vi "WID to Tree Data.vi"(11 "WID":string) -> (1 "Worker Tree Depth":i32, 2 "Alias":string, 3 "Owner WID":string)   [LabVIEW 2017, in "Application Manager.lvclass"]
uses:
  Application Manager.lvclass
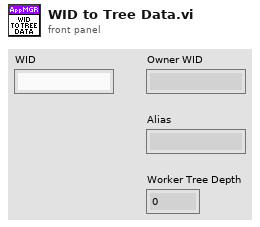
[diagram p1: front panel]
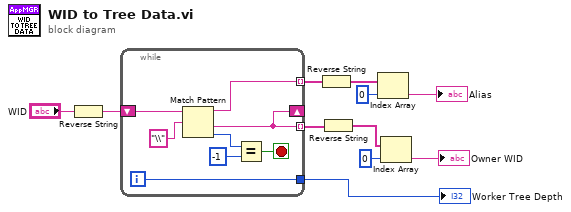
[diagram p0: block diagram]
diagram:
  n1 = Reverse String(1:"WID") -> (0:w10:string)
  n2 = while {
    shift-right: [w13] -> _
    shift-left: w10 -> [w19]
    tunnel: [w14] -> w9 mode=indexing
    tunnel: [w13] -> w3 mode=indexing
    tunnel: [w12] -> w1
    i -> [w12]
    stop <- w15 stop-if-true
    n3 = Match Pattern(string=w19, regular expression="\\") -> (before substring=w14:string, after substring=w13:string, offset past match=w17:i32)  [unwired: 1 in, 1 out]
    n4 = Equal?(x=w17, y=-1) -> (x = y?=w15:bool)
  }
  "Worker Tree Depth" <- w1
  n5 = Reverse String(1:w9) -> (0:w6:string[])
  n6 = Reverse String(1:w3) -> (0:w2:string[])
  n7 = Index Array(array=w6, index=0) -> (element=→"Alias":string)
  n8 = Index Array(array=w2, index=0) -> (element=→"Owner WID":string)
